vi "Generate Random Gene.vi"(8 "error in":errorcluster, 11 "Binary Gene in":refnum<class "Binary Gene.lvclass">) -> (0 "error out":errorcluster, 3 "Binary Gene out":refnum<class "Binary Gene.lvclass">)   [LabVIEW 2016, in "Binary Gene.lvclass"]
doc: "This VI generates a random Binary Gene allele (True or False) with probabililty of ~50% (@Normal Distribution).\nThis is an overloaded VI of IGene method.\n\n**Author: Stas Legedza"
uses:
  Binary Gene.lvclass
  C:/Users/Dzak/Documents/Projects/Evolutionary Programming/Evolutionary Programming/GA Framework/IGene/IGene.lvclass
  _typedefs/IGene_GeneType.ctl
  Binary Gene.lvclass/Binary Gene.ctl
  IGene.lvclass/IGene.ctl
  IGene.lvclass
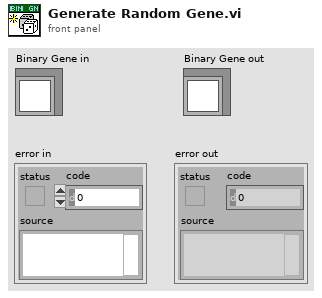
[diagram p1: front panel]
types:
  T1 = typedef "IGene.lvclass/IGene_GeneType.ctl" = enum16{"Binary", "Real", "Object", "None"}
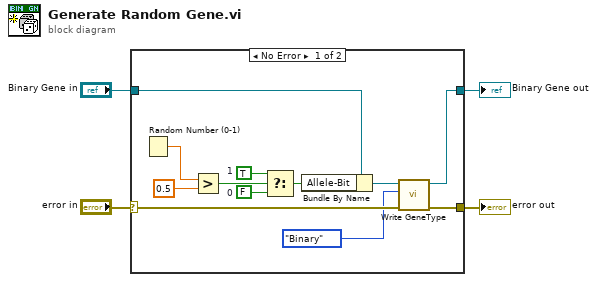
[diagram p0: block diagram]
diagram:
  n1 = case shown="No Error" "error in" {
    selector: "error in" -> [w7 w17]
    tunnel: [w8 w18] -> w4
    tunnel: "Binary Gene in" -> [w16 w18]
    tunnel: [w6 w17] -> w2
    frame No Error {
      w13 = TRUE  # 1
      w14 = FALSE  # 0
      n2 = Random Number (0-1)() -> (number: 0 to 1=w10:dbl)
      n3 = Greater?(x=w10, y=0.5) -> (0:w12:bool)
      n4 = Select(t=w13, s=w12, f=w14) -> (s? t:f=w15:bool)
      n5 = Bundle By Name(cluster=w16, "Allele-Bit"=w15) -> (w9:refnum<class "Binary Gene.lvclass">)
      n6 = call "Write GeneType.vi"("error in (no error)"=w7, "GeneType"=IGene_GeneType."Binary", "IGene in"=w9) -> ("error out"=w6:errorcluster, "IGene out"=w8:refnum<class "Binary Gene.lvclass">)  [unwired: 7 in]
    }
    frame Error {
    }
  }
  "error out" <- w2
  "Binary Gene out" <- w4
